vi "deleteTuplaEnDBEstadistica.vi"(8 "error in":errorcluster, 11 "claseEstadistica in":refnum<class "claseEstadistica.lvclass">) -> (0 "error out":errorcluster, 3 "claseEstadistica out":refnum<class "claseEstadistica.lvclass">)   [LabVIEW 2014, in "claseEstadistica.lvclass"]
uses:
  claseEstadistica.lvclass
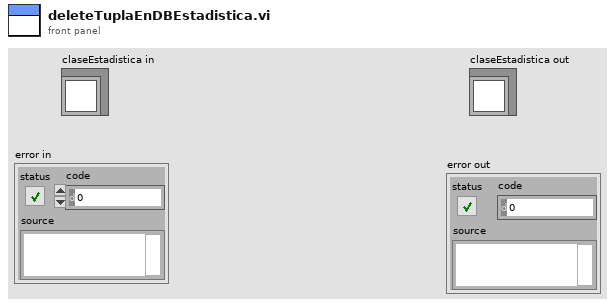
[diagram p1: front panel]
types:
  T1 = cluster{"idEstadistica":dbl, "camposDeMedicionEstadistica":string, "dateCreateEstadistica":timestamp}
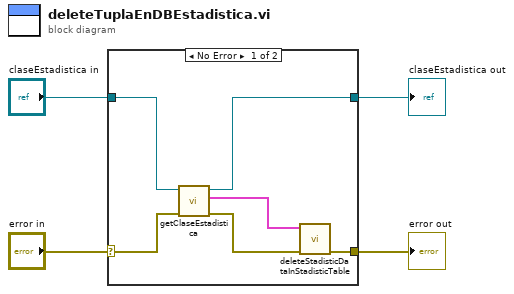
[diagram p0: block diagram]
diagram:
  n1 = case shown="No Error" "error in" {
    selector: "error in" -> [w6 w12]
    tunnel: [w5 w12] -> w3
    tunnel: [w7 w11] -> w2
    tunnel: "claseEstadistica in" -> [w10 w11]
    frame No Error {
      n2 = call "getClaseEstadistica.vi"("claseEstadistica in"=w10, "error in"=w6) -> ("claseEstadistica out"=w7:refnum<class "claseEstadistica.lvclass">, "dataReading"=w9:T1, "error out"=w8:errorcluster)  [unwired: 6 in]
      n3 = call "deleteStadisticDataInStadisticTable.vi"("error in"=w8, "dataReadingToDelete"=w9) -> ("error out"=w5:errorcluster)  [unwired: 9 in]
    }
    frame Error {
    }
  }
  "claseEstadistica out" <- w2
  "error out" <- w3
